vi "Acquire.vi"(8 "error in (no error)":errorcluster, 10 "Instrument Manager":refnum<queue>, 11 "Acquisition Config in":T1) -> (0 "error out":errorcluster, 3 "Acquisition Config out (dup)":T1)   [LabVIEW 2020, in "Omega Platinum Series Plugin.lvlib" / "Acquisition.lvlib"]
doc: "Perform the acquisition. Replace the contents of this diagram with calls to acquisition hardware."
uses:
  Acquisition.lvlib
  Hardware Configuration.ctl
  support/Message Queue/Message Cluster.ctl
  support/Message Queue/Message Queue.lvlib
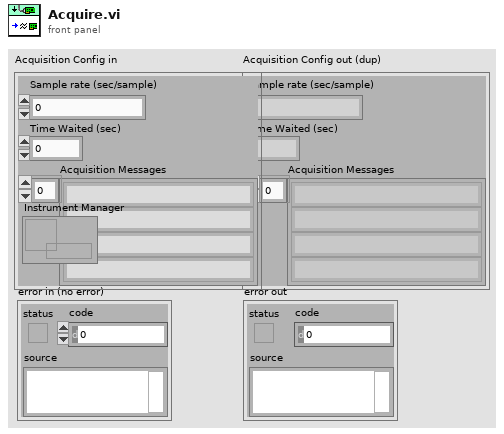
[diagram p1: front panel]
types:
  T1 = typedef "Omega Platinum Series Plugin.lvlib/Acquisition.lvlib/Hardware Configuration.ctl" = cluster{"Sample rate (sec/sample)":dbl, "Time Waited (sec)":dbl, "Acquisition Messages":string[]}
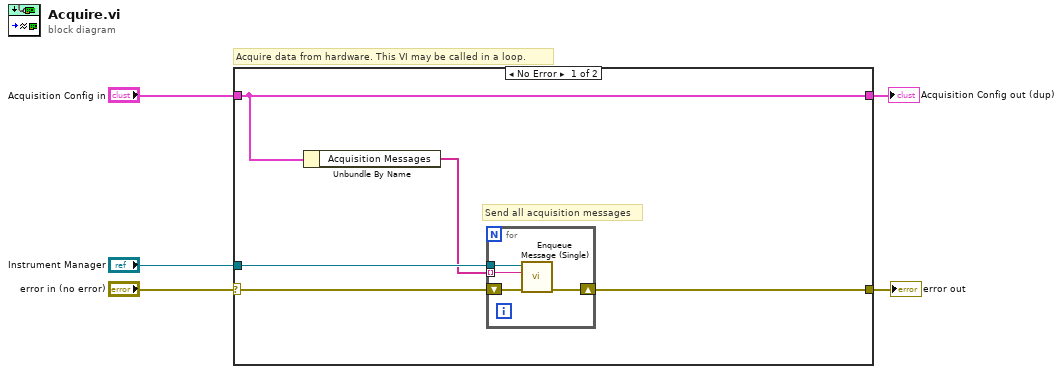
[diagram p0: block diagram]
diagram:
  # "Acquire data from hardware. This VI may be called in a loop."
  n1 = case shown="No Error" "error in (no error)" {
    selector: "error in (no error)" -> [w10 w15]
    tunnel: [w8 w15] -> w4
    tunnel: "Acquisition Config in" -> [w9 w16]
    tunnel: [w9 w16] -> w2
    tunnel: "Instrument Manager" -> [w7 _]
    frame No Error {
      # "Send all acquisition messages"
      n2 = Unbundle By Name(w9) -> ("Acquisition Messages"=w6:string[])
      n3 = for {
        tunnel: w7 -> [w12]
        shift-right: [w13] -> w8
        shift-left: w10 -> [w14]
        tunnel: w6 -> [w11] mode=indexing
        n4 = call "Enqueue Message (Single).vi"("error in (no error)"=w14, "Message"=w11, "Message Queue"=w12) -> ("error out"=w13:errorcluster)  [unwired: 7 in, 1 out]
      }
    }
    frame Error {
    }
  }
  "Acquisition Config out (dup)" <- w2
  "error out" <- w4
